vi "CheckBatteryPreProcess.vi"(0 "Image Src":T1, 11 "error in":errorcluster) -> (4 "Image Out":T1(plugin-control), 15 "error out":errorcluster)   [LabVIEW 2019]
uses:
  <vilib>/vision/Image Controls.llb/IMAQ Image.ctl
  Ctrl/UpGrayImg.ctl
  <vilib>/vision/NI_Vision_Development_Module.lvlib
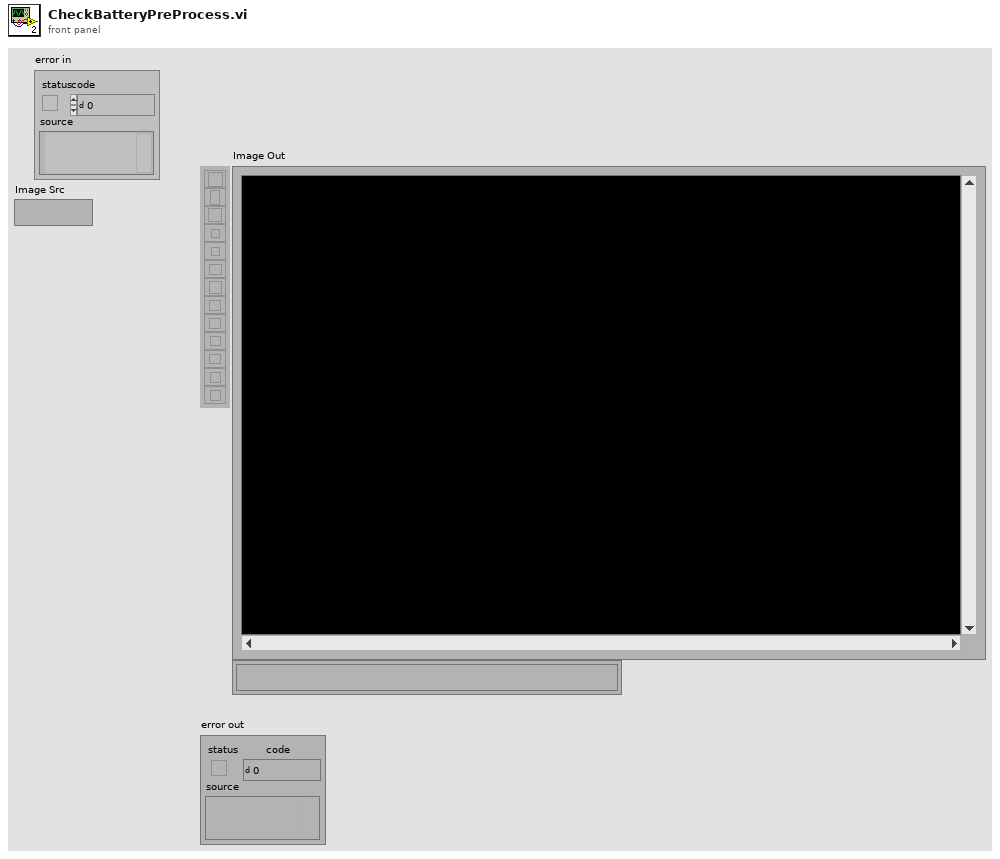
[diagram p1: front panel]
types:
  T1 = typedef "IMAQ Image.ctl" = refnum<image>
  T2 = typedef "UpGrayImg.ctl" = enum16{"CUpGray", "CUpProce1", "CUpProce2", "UpPattern1", "UpPattern2", "UpCalibImg", "UpPreProcess"}
  T3 = enum32{"AutoM", "Close", "Dilate", "Erode", "Gradient", "Gradient out", "Gradient in", "Hit miss", "Open", "PClose", "POpen", "Thick", "Thin"}
  T4 = enum32{"Linear", "Log", "Exp", "Square", "Square root", "Power X", "Power 1/X"}
  T5 = typedef "Image Type" = u32
  T6 = cluster{"histogram":u32[], "Minimal Value":sgl, "Maximal Value":sgl, "Starting Value":sgl, "Interval Width":sgl, "Mean Value":sgl, "Standard  Variation":sgl, "Area (pixels)":i32}
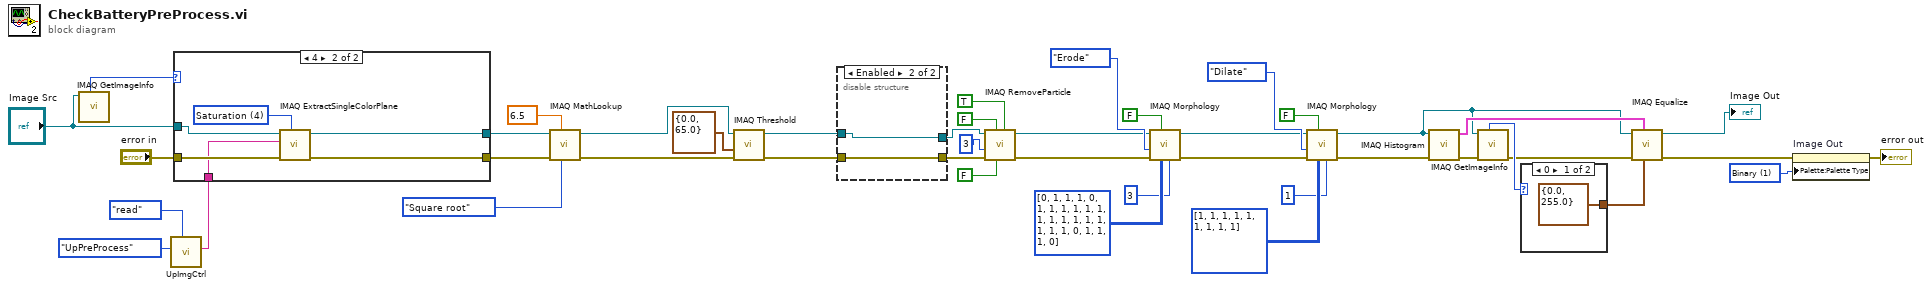
[diagram p0: block diagram]
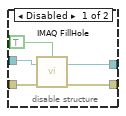
[diagram p2: hidden frame]
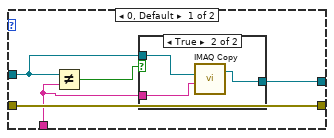
[diagram p3: hidden frame]
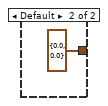
[diagram p5: hidden frame]
diagram:
  w10 = u32 1 items=["Grayscale", "Binary", "Gradient", "Rainbow", "Temperature", "User Defined", "Binary 16 Bit", "Gradient 16 Bit", "Rainbow 16 Bit", "Temperature 16 Bit", "User Defined 16 Bit"] ("Palette Type")
  n1 = call "IMAQ GetImageInfo"("Image"="Image Src") -> ("Image Type"=w7:T5)  [unwired: 3 in, 7 out]
  n2 = call "UpImgCtrl.vi"("Action"=enum16{"Initial", "read", "release"}."read", "GrayImg 2"=UpGrayImg."UpPreProcess") -> ("GrayImg"=w2:string)  [unwired: 8 in, 1 out]
  n3 = case shown="4" w7 {
    tunnel: [w49 w58] -> w44
    tunnel: [w45 w57] -> w41
    tunnel: "error in" -> [w49 w56]
    tunnel: "Image Src" -> [w48 w55]
    tunnel: w2 -> [w46 w54]
    frame 0, Default {
      n4 = Not Equal?(x=w48, y=w46) -> (x != y?=w47:bool)
      n5 = case shown="True" w47 {
        tunnel: w48 -> [w50 w53]
        tunnel: w46 -> [_ w52]
        tunnel: [w50 w51] -> w45
        frame False {
        }
        frame True {
          n6 = call "IMAQ Copy"("Image Dst"=w52, "Image Src"=w53) -> ("Image Dst Out"=w51:T1)  [unwired: 4 in, 1 out]
        }
      }
    }
    frame 4 {
      w59 = 4 items=["Red", "Green", "Blue", "Hue", "Saturation", "Luminance", "Value", "Intensity"] ("Color Plane")
      n7 = call "IMAQ ExtractSingleColorPlane"("Color Plane"=w59, "error in (no error)"=w56, "Image Dst"=w54, "Image Src"=w55) -> ("error out"=w58:errorcluster, "Image Dst Out"=w57:T1)  [unwired: 6 out]
    }
  }
  n8 = call "IMAQ MathLookup"("Operator"=T4."Square root", "X Value"=sgl 6.5, "error in (no error)"=w44, "Image Src"=w41) -> ("error out"=w40:errorcluster, "Image Dst Out"=w38:T1)  [unwired: 3 in, 3 out]
  n9 = call "IMAQ Threshold"("error in (no error)"=w40, "Range"=cluster{"Lower value":sgl, "Upper value":sgl} {"Lower value"=0.0, "Upper value"=65.0}, "Image Src"=w38) -> ("error out"=w37:errorcluster, "Image Dst Out"=w36:T1)  [unwired: 3 in, 4 out]
  n10 = disable-structure shown="Enabled" {
    disable-tunnel: w37 -> [w64 w65]
    disable-tunnel: w36 -> [w62 w66]
    disable-tunnel: [w61 w65] -> w35
    disable-tunnel: [w60 w66] -> w31
    frame Disabled {
      n11 = call "IMAQ FillHole"("error in (no error)"=w64, "Image Src"=w62, "Connectivity 4/8 (8)"=TRUE) -> ("error out"=w61:errorcluster, "Image Dst Out"=w60:T1)  [unwired: 1 in, 2 out]
    }
    frame Enabled {
    }
  }
  n12 = call "IMAQ RemoveParticle"("Connectivity 4/8 (8)"=TRUE, "Low Pass/High Pass (Low)"=FALSE, "Square/Hexa (Square)"=FALSE, "error in (no error)"=w35, "Number of Erosion"=3, "Image Src"=w31) -> ("error out"=w30:errorcluster, "Image Dst Out"=w25:T1)  [unwired: 1 in, 3 out]
  n13 = call "IMAQ Morphology"("Number of iterations (1)"=3, "Structuring Element"=i32[][] [[0, 1, 1, 1, 0], [1, 1, 1, 1, 1], [1, 1, 1, 1, 1], [1, 1, 1, 1, 1], [0, 1, 1, 1, 0]], "Square/Hexa (Square)"=FALSE, "error in (no error)"=w30, "Operation"=T3."Erode", "Image Src"=w25) -> ("error out"=w24:errorcluster, "Image Dst Out"=w19:T1)  [unwired: 1 in, 3 out]
  n14 = call "IMAQ Morphology"("Number of iterations (1)"=1, "Structuring Element"=i32[][] [[1, 1, 1], [1, 1, 1], [1, 1, 1]], "Square/Hexa (Square)"=FALSE, "error in (no error)"=w24, "Operation"=T3."Dilate", "Image Src"=w19) -> ("error out"=w18:errorcluster, "Image Dst Out"=w15:T1)  [unwired: 1 in, 3 out]
  n15 = call "IMAQ Histogram"("error in (no error)"=w18, "Image"=w15) -> ("error out"=w14:errorcluster, "Histogram Report"=w17:T6)  [unwired: 3 in, 5 out]
  n16 = call "IMAQ GetImageInfo"("error in (no error)"=w14, "Image"=w15) -> ("error out"=w13:errorcluster, "Image Type"=w16:T5)  [unwired: 8 out]
  n17 = case shown="0" w16 {
    tunnel: [cluster{"Minimum":sgl, "Maximum":sgl} {"Minimum"=0.0, "Maximum"=255.0} ("Range") cluster{"Minimum":sgl, "Maximum":sgl} {"Minimum"=0.0, "Maximum"=0.0} ("Range")] -> w12
    frame 0 {
    }
    frame Default {
    }
  }
  n18 = call "IMAQ Equalize"("Range"=w12, "Histogram Report"=w17, "error in (no error)"=w13, "Image Src"=w15) -> ("error out"=w6:errorcluster, "Image Dst Out"=→"Image Out":T1)  [unwired: 2 in, 4 out]
  n19 = property on="Image Out" class="ImageControl"(error in=w6, "Palette:Palette Type"=w10) -> (error out=→"error out":errorcluster)  [unwired: 1 in, 1 out]
